vi "Echo Response.vi"(8 "error in (no error)":errorcluster, 11 "Port Selection Info":T1={"Port Name"="", "Amplifier Num"=1, "Baud Rate"=38400, "Char Formation"=enum."0"} {"Baud Rate" items=["38400"=38400, "19200"=19200, "9600"=9600, "115200"=0]; "Amplifier Num" max=31}) -> (0 "error out":errorcluster, 1 "Info Code":u16 format="%.0x", 2 "Info Data":u16 format="%.0x", 3 "Port Selection Info Out":T1={"Port Name"="", "Amplifier Num"=1, "Baud Rate"=38400, "Char Formation"=enum."0"} {"Baud Rate" items=["38400"=38400, "19200"=19200, "9600"=9600, "115200"=0]; "Amplifier Num" max=31}, 4 "Check Result":bool, 5 "FC":u8, 6 "Bytes Received":u32, 7 "Amplifier Num":u8)   [LabVIEW 2014, in "ALPHA5 RS485.lvlib"]
uses:
  ALPHA5 RS485.lvlib
  typedefs/Port Selection Info.ctl
panel:
  # "Wait for at least 15ms after sending out  echo test command."
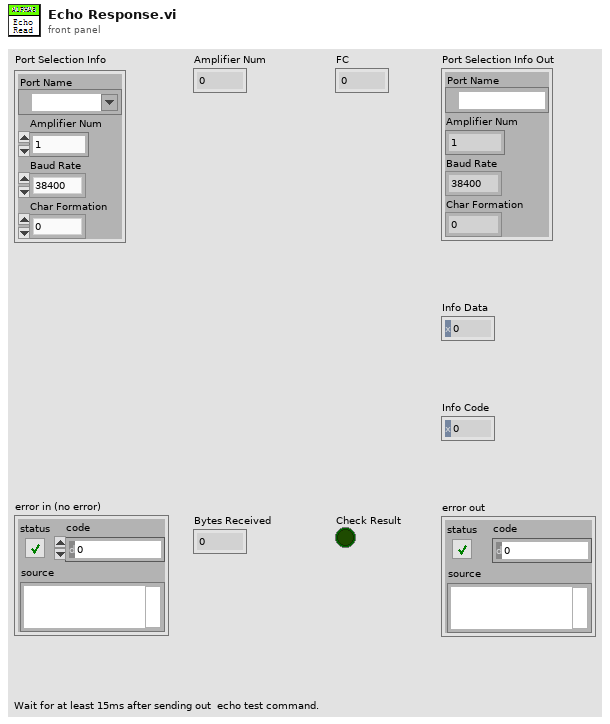
[diagram p1: front panel]
types:
  T1 = typedef "ALPHA5 RS485.lvlib/Port Selection Info.ctl" = cluster{"Port Name":refnum<visa-resource-name>, "Amplifier Num":u8, "Baud Rate":u32, "Char Formation":enum16{"0", "1", "2", "3", "4", "5"}}
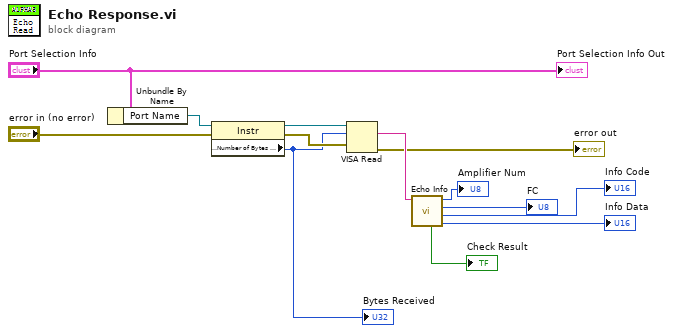
[diagram p0: block diagram]
diagram:
  n1 = Unbundle By Name("Port Selection Info") -> ("Port Name"=w7:refnum<visa-resource-name>)
  n2 = property class="Instr"(reference=w7, error in="error in (no error)") -> (reference out=w6:refnum<visa-resource-name>, error out=w8:errorcluster, "Serial Settings:Number of Bytes at Serial Port"=w1:u32)
  "Bytes Received" <- w1
  n3 = VISA Read(VISA resource name=w6, byte count=w1, error in (no error)=w8) -> (read buffer=w12:string, error out=→"error out":errorcluster)  [unwired: 2 out]
  n4 = call "Echo Info.vi"("Echo Info"=w12) -> ("Info Data"=→"Info Data":u16, "Info Code"=→"Info Code":u16, "FC"=→"FC":u8, "Amplifier Num"=→"Amplifier Num":u8, "Check Result"=→"Check Result":bool)  [unwired: 6 in]
  "Port Selection Info Out" <- "Port Selection Info"
